vi "dispense exercise.vi"() -> ()   [LabVIEW 2016]
uses:
  Classes/Controller/Dispenser/Ultimus V2 Folder/Ultimus V2.lvclass
panel:
  out ".not. (x .xor. y)?":bool
  in  "x":bool
  in  "y":bool
  in  "Delay Time (s)":dbl=0.1
  in  "stop":bool
  in  "run":bool
  in  "change status":bool
  in  "Vacuum Setting (0000)":i64 min=0 max=1000 step=1 format="%04.0f"
  in  "Pressure":i16
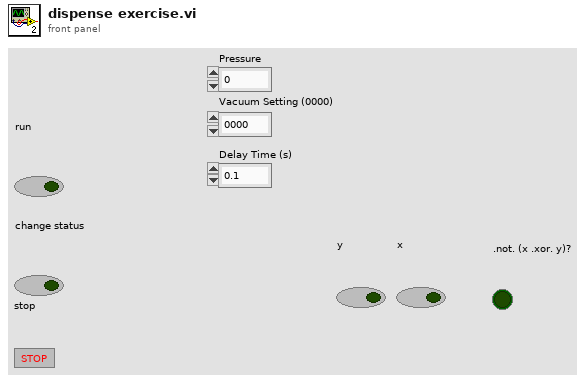
[diagram p1: front panel]
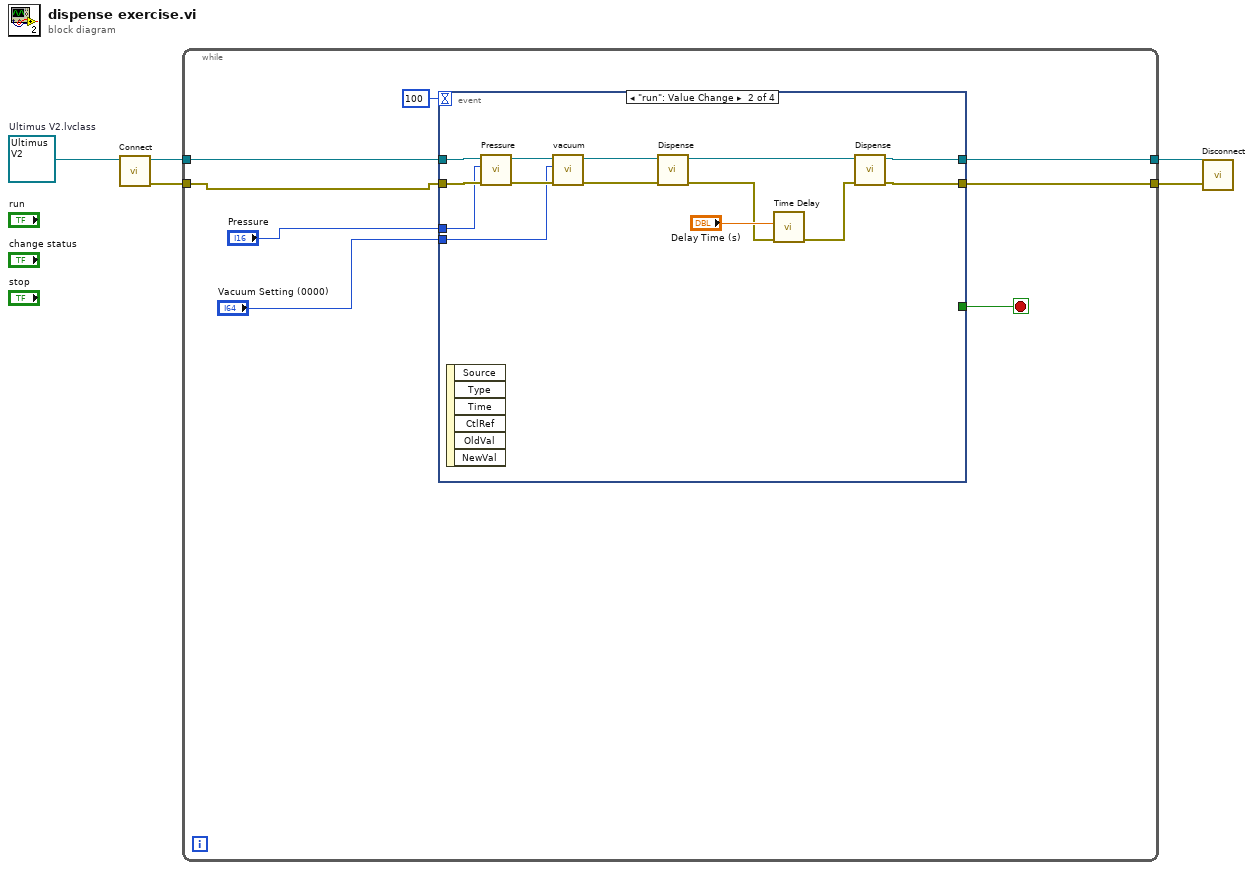
[diagram p0: block diagram]
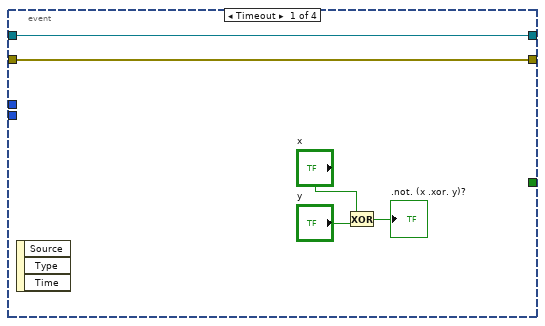
[diagram p2: hidden frame]
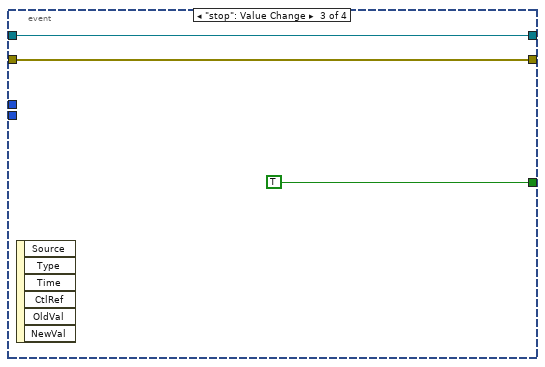
[diagram p3: hidden frame]
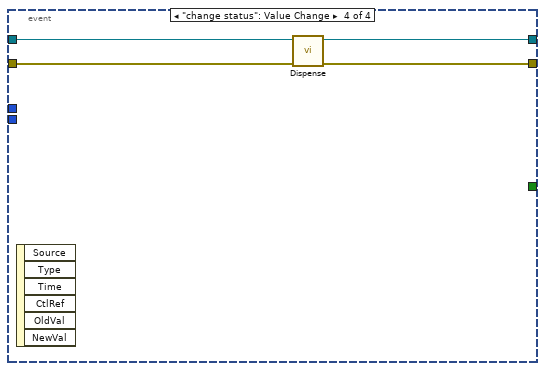
[diagram p4: hidden frame]
diagram:
  w4 = refnum<class "Ultimus V2.lvclass"> refnum  # Ultimus V2.lvclass
  n1 = call-dynamic "Connect.vi"("Ultimus V in"=w4) -> ("error out"=w2:errorcluster, "Ultimus V out"=w3:refnum<class "Ultimus V2.lvclass">)  [unwired: 9 in]
  n2 = while {
    tunnel: [w13] -> w5
    tunnel: w3 -> [w7]
    tunnel: w2 -> [w6]
    tunnel: [w12] -> w1
    stop <- w11 stop-if-true
    n3 = event shown="[1] \"run\": Value Change" {
      selector: _ -> [_ _ _ _]
      dyn-events: _ -> [_ _ _ _]
      timeout: 100 -> [_ _ _ _]
      tunnel: w7 -> [w17 w21 w33 w39]
      tunnel: [w17 w31 w33 w36] -> w13
      tunnel: w6 -> [w18 w26 w34 w38]
      tunnel: [w18 w32 w34 w37] -> w12
      tunnel: [_ _ TRUE _] -> w11
      tunnel: "Vacuum Setting (0000)" -> [_ w20 _ _]
      tunnel: "Pressure" -> [_ w19 _ _]
      event Timeout {
        n4 = event-data() -> ()  [unwired: 1 in, 3 out]
        n5 = Exclusive Or(1:"y", 2:"x") -> (0:→".not. (x .xor. y)?":bool)
      }
      event "run": Value Change {
        n6 = event-data() -> ()  [unwired: 1 in, 6 out]
        n7 = call-dynamic "Pressure.vi"("error in (no error)"=w26, "Pressure"=w19, "Ultimus V in"=w21) -> ("error out"=w25:errorcluster, "Ultimus V out"=w22:refnum<class "Ultimus V2.lvclass">)  [unwired: 7 in]
        n8 = call "vacuum.vi"("error in (no error)"=w25, "Vacuum Setting (0000)"=w20, "Ultimus V in"=w22) -> ("error out"=w24:errorcluster, "Ultimus V out"=w23:refnum<class "Ultimus V2.lvclass">)  [unwired: 7 in]
        n9 = call-dynamic "Dispense.vi"("error in (no error)"=w24, "Ultimus V in"=w23) -> ("error out"=w28:errorcluster, "Ultimus V out"=w30:refnum<class "Ultimus V2.lvclass">)  [unwired: 8 in]
        n10 = call "Time Delay"("error in (no error)"=w28, "Delay Time (s)"="Delay Time (s)") -> ("error out"=w27:errorcluster)  [unwired: 9 in]
        n11 = call-dynamic "Dispense.vi"("error in (no error)"=w27, "Ultimus V in"=w30) -> ("error out"=w32:errorcluster, "Ultimus V out"=w31:refnum<class "Ultimus V2.lvclass">)  [unwired: 8 in]
      }
      event "stop": Value Change {
        n12 = event-data() -> ()  [unwired: 1 in, 6 out]
      }
      event "change status": Value Change {
        n13 = event-data() -> ()  [unwired: 1 in, 6 out]
        n14 = call-dynamic "Dispense.vi"("error in (no error)"=w38, "Ultimus V in"=w39) -> ("error out"=w37:errorcluster, "Ultimus V out"=w36:refnum<class "Ultimus V2.lvclass">)  [unwired: 8 in]
      }
    }
  }
  n15 = call-dynamic "Disconnect.vi"("error in (no error)"=w1, "Ultimus V in"=w5) -> ()  [unwired: 8 in, 1 out]
